vi "stop_FGV.vi"(7 "comandos":enum16{"Iniciar", "Parar", "Parar?"}(ring)=enum."Parar?", 8 "error in":errorcluster) -> (0 "error out":errorcluster, 4 "parar?":bool)   [LabVIEW 2018]
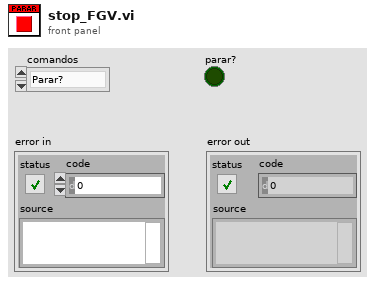
[diagram p1: front panel]
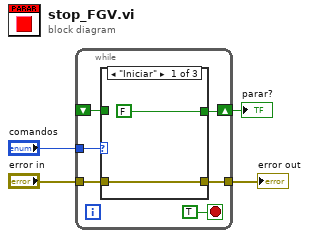
[diagram p0: block diagram]
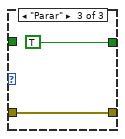
[diagram p3: hidden frame]
diagram:
  n1 = while {
    tunnel: "error in" -> [w6]
    tunnel: [w5] -> w1
    tunnel: "comandos" -> [w9]
    shift-right: [w8] -> w3
    shift-left: _ -> [w7]
    stop <- TRUE stop-if-true
    n2 = case shown="\"Iniciar\"" w9 {
      tunnel: [FALSE w13 TRUE] -> w8
      tunnel: w7 -> [_ w13 _]
      tunnel: w6 -> [w11 w14 w15]
      tunnel: [w11 w14 w15] -> w5
      frame "Iniciar" {
      }
      frame "Parar?", Default {
      }
      frame "Parar" {
      }
    }
  }
  "error out" <- w1
  "parar?" <- w3
